vi "Do while loop.vi"() -> ()   [LabVIEW 2023]
panel:
  out "size(s) 2":i32
  out "size(s)":i32
  out "Array 2":dbl[](array[numeric])
  out "Array":dbl[](array[numeric])
  # "While 循环"
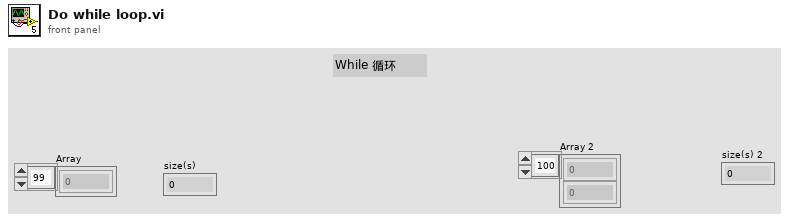
[diagram p1: front panel]
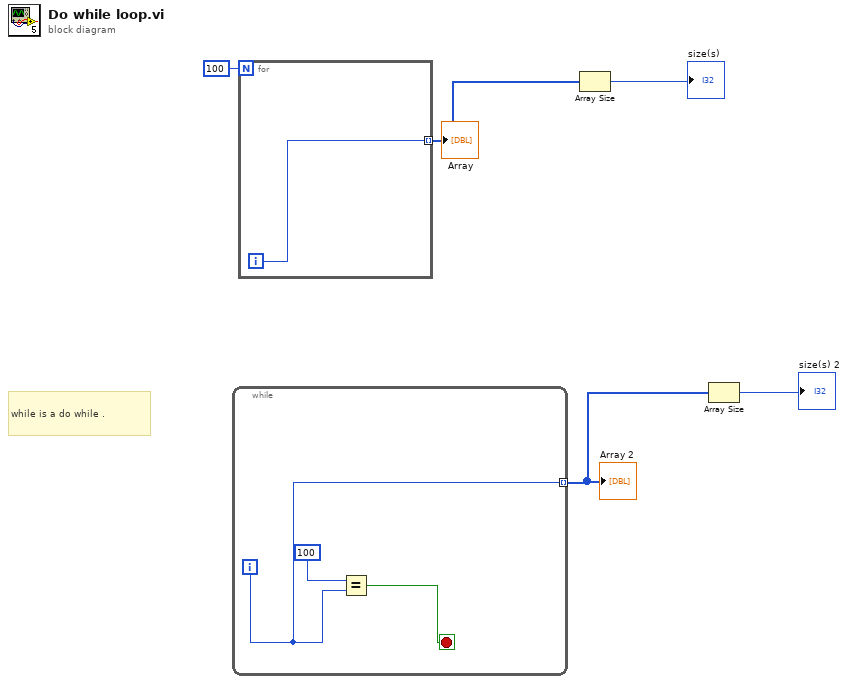
[diagram p0: block diagram]
diagram:
  # "while is a do while ."
  n1 = while {
    tunnel: [w6] -> w2 mode=indexing
    i -> [w6]
    stop <- w7 stop-if-true
    n2 = Equal?(x=100, y=w6) -> (x = y?=w7:bool)
  }
  "Array 2" <- w2
  n3 = for {
    N: 100 -> [_]
    tunnel: [w9] -> w4 mode=indexing
    i -> [w9]
  }
  "Array" <- w4
  n4 = Array Size(array=w4) -> (size(s)=→"size(s)":i32)
  n5 = Array Size(array=w2) -> (size(s)=→"size(s) 2":i32)
